vi "Message encoder.vi"(8 "error in (no error)":errorcluster, 10 "Data":variant, 11 "TCP Writer in":refnum<class "TCP Writer.lvclass">) -> (0 "error out":errorcluster, 2 "Message encoded":string, 3 "TCP Writer out":refnum<class "TCP Writer.lvclass">)   [LabVIEW 2026, in "TALOS.lvlib" / "TCP Writer.lvlib" / "TCP Writer.lvclass"]
uses:
  TCP Writer.lvclass
  TCP Message.ctl
  Ancestor/Ancestor/Ancestor.lvclass/Ancestor.ctl
  Support VIs/Generate Error.vi
  FGV/Error Memory/Get Error Description.vi
  Support VIs/Get PC name.vi
  Ancestor/Ancestor/Read ID.vi
  Support VIs/Get Class Name.vi
  <vilib>/Utility/error.llb/Clear Errors.vi
  FGV/Error Memory/Error Memory Core.vi
  <vilib>/AdvancedString/Delimited String to 1D String Array.vi
  <vilib>/AdvancedString/Delimited String to 1D String Array (string).vi
  Support VIs/Circus Root Path.vi
  FGV/Error Memory/Error Crt Lvl checker.vi
  FGV/Error Memory/Error Memory Core.vi/40c8088d-b597-4017-91af-faa98e00292e.vi
  FGV/Error Memory/Error Memory Core.vi/d4a3ab98-063c-4e44-b43d-fbdcfe6c2be2.vi
  Support VIs/Global Memory.vi
  <vilib>/Utility/LVClass/Get LV Class Name.vi
  Support VIs/Is in Packed Library.vi
  Support VIs/TALOS Root path.vi
  Support VIs/Read CSV worksheet.vi
  Support VIs/Global Constants.vi
  <vilib>/Utility/error.llb/General Error Handler.vi
  Support VIs/Error Log.vi
  Ancestor/Ancestor/Ancestor.lvclass
  <vilib>/Comparison/Equal/Equal Functor/Equal Functor.lvclass
  TALOS.lvlib
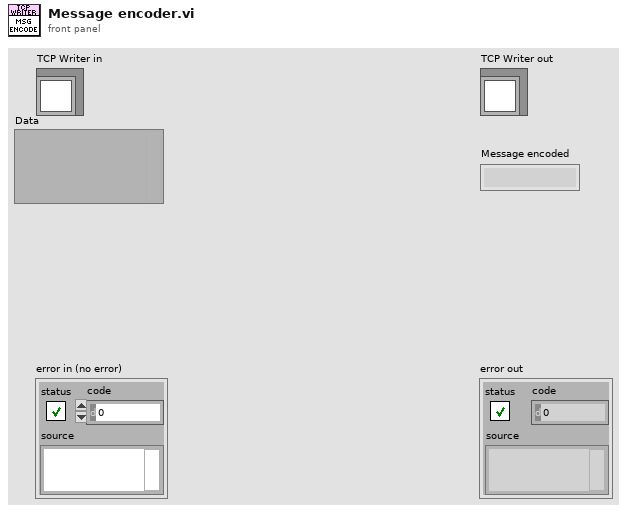
[diagram p1: front panel]
types:
  T1 = typedef "TALOS.lvlib/TCP Writer.lvlib/TCP Writer.lvclass/TCP Message.ctl" = cluster{"Type string":i16[], "Data string":string}
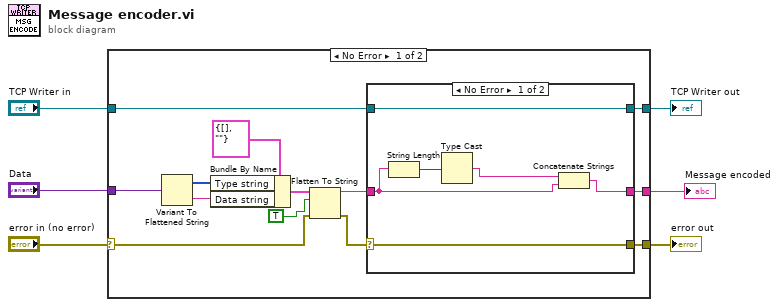
[diagram p0: block diagram]
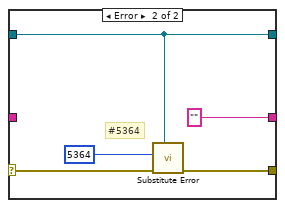
[diagram p2: hidden frame]
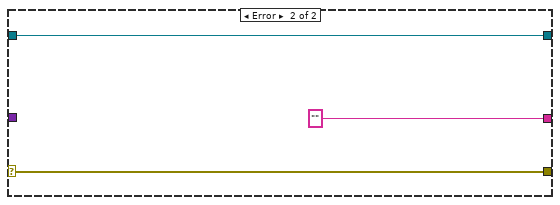
[diagram p3: hidden frame]
diagram:
  n1 = case shown="No Error" "error in (no error)" {
    selector: "error in (no error)" -> [w18 w33]
    tunnel: [w11 w33] -> w5
    tunnel: [w15 w32] -> w3
    tunnel: "TCP Writer in" -> [w14 w32]
    tunnel: [w12 "" ("data string")] -> w2
    tunnel: "Data" -> [w17 _]
    frame No Error {
      n2 = Variant To Flattened String(Variant=w17) -> (data string=w8:string, 1:w9:i16[])
      n3 = Bundle By Name(cluster=T1 {"Type string"=[], "Data string"=""}, "Type string"=w9, "Data string"=w8) -> (w19:T1)
      n4 = Flatten To String(anything=w19, prepend array or string size? (T)=TRUE, error in (no error)=w18) -> (data string=w13:string, error out=w16:errorcluster)  [unwired: 1 in, 1 out]
      n5 = case shown="No Error" w16 {
        selector: w16 -> [w21 w28]
        tunnel: [w25 w29] -> w15
        tunnel: w14 -> [w25 w29]
        tunnel: w13 -> [w23 _]
        tunnel: [w22 ""] -> w12
        tunnel: [w21 w27] -> w11
        frame No Error {
          n6 = String Length(string=w23) -> (length=w20:i32)
          n7 = Type Cast(x=w20) -> (*(type *) &x=w24:string)  [unwired: 1 in]
          n8 = Concatenate Strings(w24, w23) -> (w22:string)
        }
        frame Error {
          # "#5364"
          n9 = call "Substitute Error.vi"("LabVIEW Object"=w29, "error in (no error)"=w28, "Error Code"=5364) -> ("error out"=w27:errorcluster)  [unwired: 8 in]
        }
      }
    }
    frame Error {
    }
  }
  "error out" <- w5
  "TCP Writer out" <- w3
  "Message encoded" <- w2
